vi "Save As Fits.vi"(8 "error in (no error)":errorcluster, 11 "CCDCamera in":refnum<class "CCDCamera.lvclass">) -> (0 "error out":errorcluster, 3 "CCDCamera out":refnum<class "CCDCamera.lvclass">)   [LabVIEW 2018, in "CCDCamera.lvclass"]
doc: "This VI reads the last image, image path, and the FITS format to save the last acquisition."
uses:
  CCDCamera.lvclass
  CCDCamera.lvclass/CCDCamera.ctl
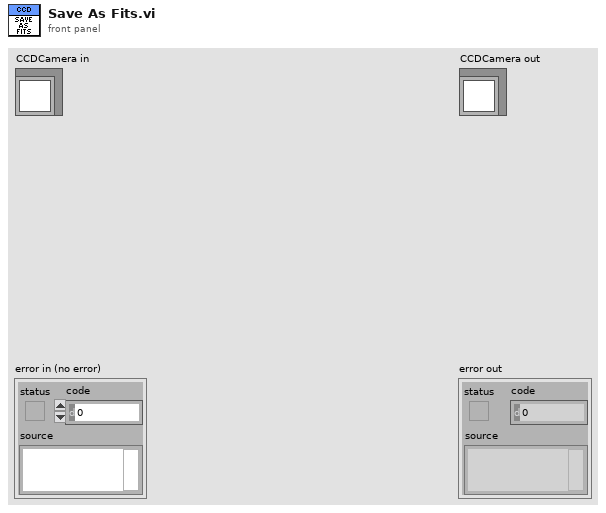
[diagram p1: front panel]
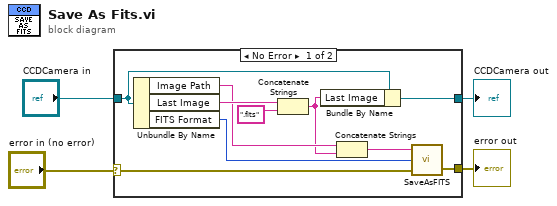
[diagram p0: block diagram]
diagram:
  n1 = case shown="No Error" "error in (no error)" {
    selector: "error in (no error)" -> [w12 w16]
    tunnel: [w13 w16] -> w3
    tunnel: [w9 w15] -> w1
    tunnel: "CCDCamera in" -> [w10 w15]
    frame No Error {
      n2 = Unbundle By Name(w10) -> ("Image Path"=w7:string, "Last Image"=w8:string, "FITS Format"=w14:u16)
      n3 = Concatenate Strings(w8, ".fits") -> (w6:string)
      n4 = Bundle By Name(cluster=w10, "Last Image"=w6) -> (w9:refnum<class "CCDCamera.lvclass">)
      n5 = Concatenate Strings(w7, w6) -> (w5:string)
      n6 = call <userlib>:"SaveAsFITS.vi"("error in (no error)"=w12, "FITS_type"=w14, "path"=w5) -> ("error out"=w13:errorcluster)  [unwired: 1 out]
    }
    frame Error {
    }
  }
  "error out" <- w3
  "CCDCamera out" <- w1
